vi "time parse and tokenize process.vi"() -> ()   [LabVIEW 2014]
uses:
  json token.ctl
  json node type.ctl
panel:
  out "values":variant[](array[variant])
  out "names":string[](array[string])
  out "variant out":variant
  out "remaining tokens":T1[](array[typedef])
  out "element":bool
  out "x-y":dbl=1.9602011889219284e-06
  in  "String":string="{\n    \"id\": 1,\n    \"name\": \"Foo\",\n    \"price\": 123,\n    \"tags\": [ \"Bar\", \"Eek\" ],\n    \"stock\": {\n        \"warehouse\": 300,\n        \"retail\": 20\n    }\n}"
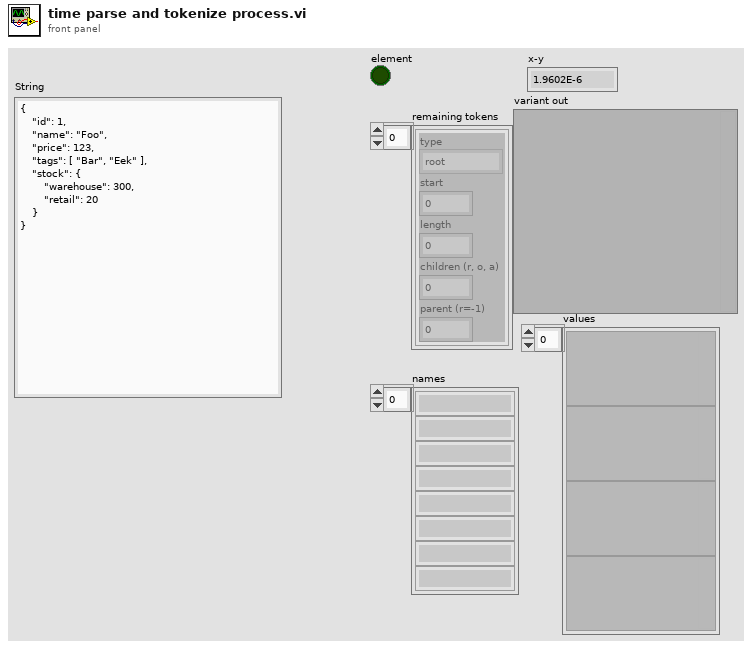
[diagram p1: front panel]
types:
  T1 = typedef "json token.ctl" = cluster{"type":T2, "start":i32, "length":i32, "children (r, o, a)":u16, "parent (r=-1)":i32}
  T2 = typedef "json node type.ctl" = enum16{"root", "object", "array", "number", "string value", "string key", "true", "false", "null"}
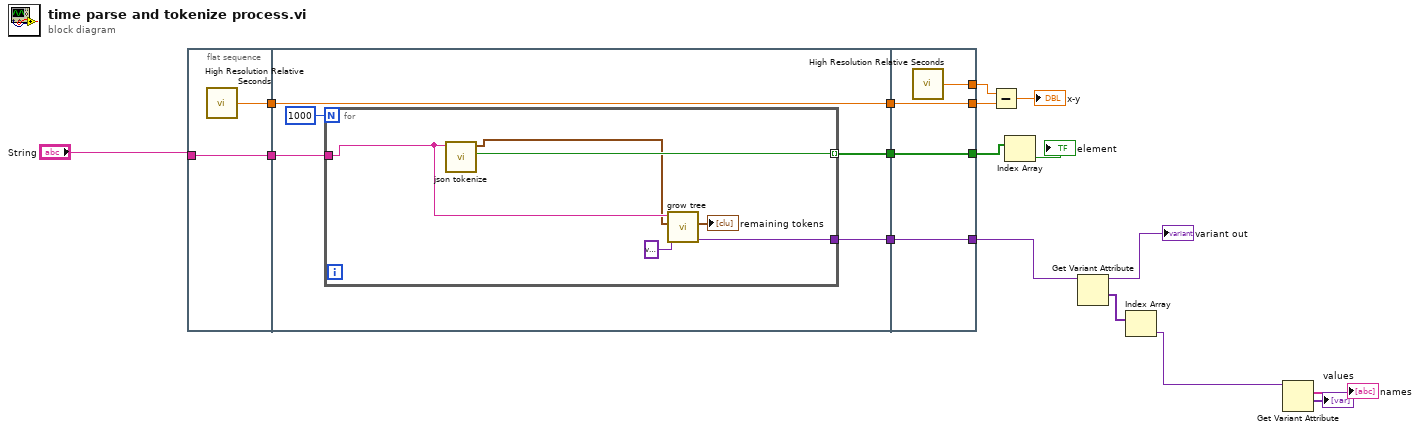
[diagram p0: block diagram]
diagram:
  n1 = flat-sequence {
    tunnel: "String" -> [w19]
    tunnel: [w19] -> w17
    tunnel: [w18] -> w15
    tunnel: w17 -> [w24]
    tunnel: w15 -> [w23]
    tunnel: [w23] -> w14
    tunnel: [w22] -> w9
    tunnel: [w20] -> w7
    tunnel: [w34] -> w16
    tunnel: w14 -> [w33]
    tunnel: [w33] -> w13
    tunnel: [w32] -> w10
    tunnel: w9 -> [w32]
    tunnel: [w31] -> w5
    tunnel: w7 -> [w31]
    frame #0 {
      n2 = call <vilib>:"High Resolution Relative Seconds.vi"() -> ("relative seconds"=w18:dbl)
    }
    frame #1 {
      n3 = for {
        N: 1000 ("Numeric") -> [_]
        tunnel: w24 -> [w29]
        tunnel: [w30] -> w22 mode=indexing
        tunnel: [w25] -> w20
        n4 = call "json tokenize.vi"("String"=w29) -> ("error"=w30:bool, "tokens"=w28:T1[])  [unwired: 9 in]
        n5 = call "grow tree.vi"("variant in"=variant, "tokens"=w28, "String"=w29) -> ("variant out"=w25:variant, "remaining tokens"=→"remaining tokens":T1[])  [unwired: 7 in]
      }
    }
    frame #2 {
      n6 = call <vilib>:"High Resolution Relative Seconds.vi"() -> ("relative seconds"=w34:dbl)
    }
  }
  n7 = Subtract(x=w16, y=w13) -> (x-y=→"x-y":dbl)
  n8 = Index Array(array=w10) -> (element=→"element":bool)  [unwired: 1 in]
  n9 = Get Variant Attribute(Variant=w5) -> (duplicate Variant=→"variant out":variant, values=w4:variant[])  [unwired: 3 in, 2 out]
  n10 = Index Array(array=w4) -> (element=w1:variant)  [unwired: 1 in]
  n11 = Get Variant Attribute(Variant=w1) -> (names=→"names":string[], values=→"values":variant[])  [unwired: 3 in, 2 out]
